vi "Get Available Channels.vi"(8 "error in (no error)":errorcluster, 11 "SLSC Switch in":refnum<class "SLSC Switch.lvclass">) -> (0 "error out":errorcluster, 2 "Channels":string[](array[string]), 3 "SLSC Switch out":refnum<class "SLSC Switch.lvclass">)   [LabVIEW 2015, in "SLSC Switch.lvlib" / "SLSC Switch.lvclass"]
doc: "Returns a list of all user-enabled channels available in the currently loaded topology."
uses:
  SLSC Switch.lvclass
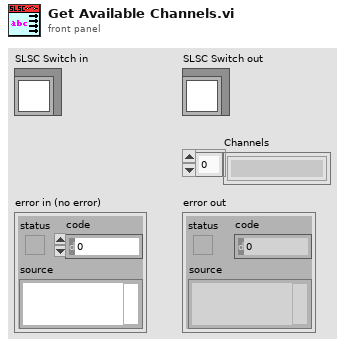
[diagram p1: front panel]
types:
  T1 = typedef "SLSC Switch.lvlib/SLSC Switch.lvclass/Topology.ctl" = cluster{"name":string, "InitialState":T2, "ChannelList":T3, "ConnectionList":T4[], "MuxList":cluster{"Src":string, "Dests":string[]}[]}
  T2 = typedef "SLSC Switch.lvlib/SLSC Switch.lvclass/JSON.InitialState.ctl" = cluster{"Open":string[], "Close":string[]}
  T3 = typedef "SLSC Switch.lvlib/SLSC Switch.lvclass/JSON.ChannelList.ctl" = cluster{"Names":string[]}
  T4 = typedef "SLSC Switch.lvlib/SLSC Switch.lvclass/JSON.ConnectionList.ctl" = cluster{"Src":string, "Dest":string, "Relays":string[]}
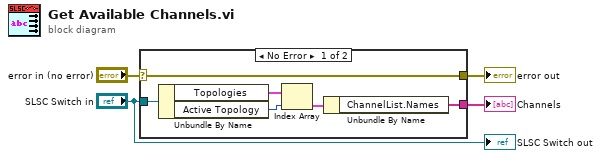
[diagram p0: block diagram]
diagram:
  n1 = case shown="No Error" "error in (no error)" {
    selector: "error in (no error)" -> [w5 w11]
    tunnel: [w5 w11] -> w3
    tunnel: [w10 _] -> w2
    tunnel: "SLSC Switch in" -> [w9 _]
    frame No Error {
      n2 = Unbundle By Name(w9) -> ("Topologies"=w8:T1[], "Active Topology"=w7:i32)
      n3 = Index Array(array=w8, index=w7) -> (element=w6:T1)
      n4 = Unbundle By Name(w6) -> ("ChannelList.Names"=w10:string[])
    }
    frame Error {
    }
  }
  "error out" <- w3
  "Channels" <- w2
  "SLSC Switch out" <- "SLSC Switch in"
